vi "Select Random Extreme Array Index.vi"(0 "Array":i32[](array[numeric])) -> (14 "Chosen Max Index":i32, 15 "Max Value":i32, 16 "Max[]":i32[](array[numeric]), 17 "Chosen Min Index":i32, 18 "Min Value":i32)   [LabVIEW 2014]
uses:
  <userlib>/_OpenG.lib/array/array.llb/Filter 1D Array with Scalar (I32)__ogtk.vi
  Dragon Tamers.lvlib
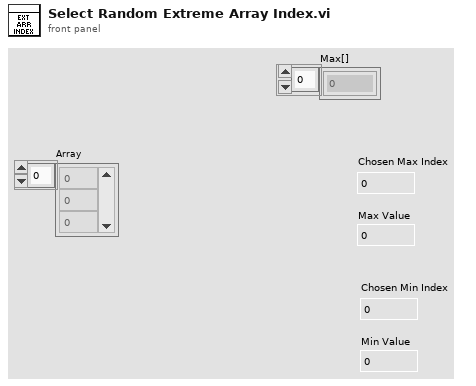
[diagram p1: front panel]
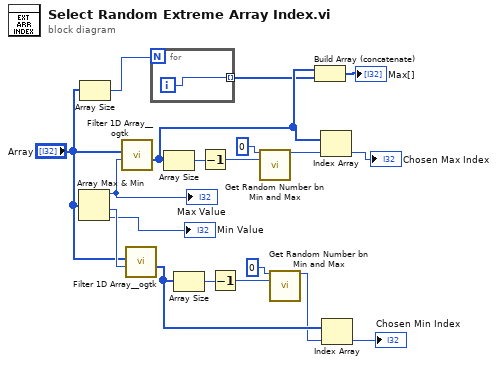
[diagram p0: block diagram]
diagram:
  n1 = Array Max & Min(array="Array") -> (max value=w19:i32, min value=w15:i32, min index (indices)=→"Min Value":i32)  [unwired: 1 out]
  "Max Value" <- w19
  n2 = Array Size(array="Array") -> (size(s)=w4:i32)
  n3 = call-poly <userlib>:"Filter 1D Array__ogtk.vi"("items to filter"=w19, "array"="Array") -> ("filtered item indices"=w3:i32[])  [unwired: 4 in, 1 out]
  n4 = call-poly <userlib>:"Filter 1D Array__ogtk.vi"("items to filter"=w15, "array"="Array") -> ("filtered item indices"=w8:i32[])  [unwired: 4 in, 1 out]
  n5 = for {
    N: w4 -> [_]
    tunnel: [w20] -> w2 mode=indexing
    i -> [w20]
  }
  n6 = Array Size(array=w3) -> (size(s)=w18:i32)
  n7 = Array Size(array=w8) -> (size(s)=w11:i32)
  n8 = Decrement(x=w18) -> (x-1=w16:i32)
  n9 = Decrement(x=w11) -> (x-1=w13:i32)
  n10 = call "Get Random Number bn Min and Max.vi"("Min"=0, "Max"=w16) -> ("Random Value"=w10:i32)  [unwired: 13 in]
  n11 = call "Get Random Number bn Min and Max.vi"("Min"=0, "Max"=w13) -> ("Random Value"=w7:i32)  [unwired: 13 in]
  n12 = Build Array (concatenate)(w3, w2) -> (→"Max[]":i32[])
  n13 = Index Array(array=w3, index=w10) -> (element=→"Chosen Max Index":i32)
  n14 = Index Array(array=w8, index=w7) -> (element=→"Chosen Min Index":i32)
